vi "WriteCurrent.vi"(10 "Current":dbl, 11 "address string in":string) -> (3 "address string in 2":string)   [LabVIEW 2017]
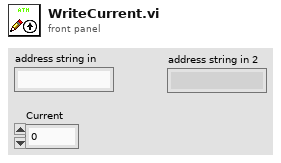
[diagram p1: front panel]
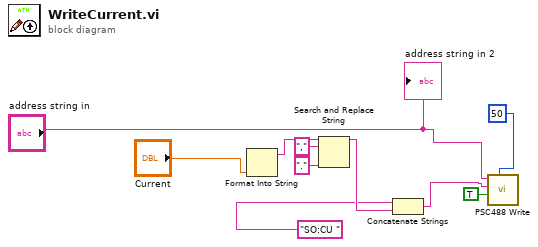
[diagram p0: block diagram]
diagram:
  n1 = Format Into String("Current") -> (resulting string=w6:string)  [unwired: 3 in, 1 out]
  n2 = Search and Replace String(input string=w6, search string=",", replace string="." ("replace string (\"\")")) -> (result string=w9:string)  [unwired: 5 in, 3 out]
  n3 = Concatenate Strings("SO:CU " ("Command"), w9) -> (w3:string)
  n4 = call "PSC488 Write.vi"("Address"="address string in", "Command"=w3, "Enable"=TRUE, "Delay after write"=u16 50) -> ()  [unwired: 1 in, 1 out]
  "address string in 2" <- "address string in"
